vi "保存历史波形图.vi"(4 "接受协议数组":T1(array[cluster]), 6 "Chart legend":T2(array[cluster]), 7 "保存开始":bool, 8 "错误输入":errorcluster, 9 "队列元素":dbl[](array[numeric]), 10 "输入":enum16{"检测按键", "设置路径", "保存数据", "关闭TDMS"}(ring), 11 "tdms file in":refnum<k34>) -> (0 "错误输出":errorcluster, 2 "输出":enum16{"检测按键", "设置路径", "保存数据", "关闭TDMS"}(ring), 3 "tdms file out":refnum<k34>)   [LabVIEW 2016]
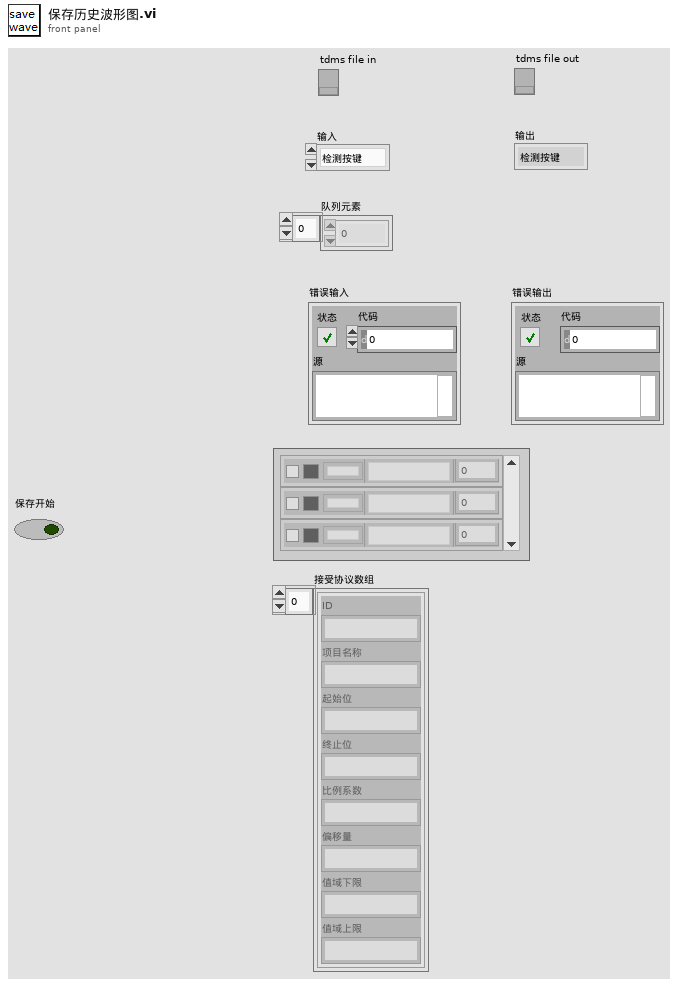
[diagram p1: front panel]
types:
  T1 = cluster{"ID":string, "项目名称":string, "起始位":string, "终止位":string, "比例系数":string, "偏移量":string, "值域下限":string, "值域上限":string}[]
  T2 = cluster{"曲线名称":string, "曲线颜色":u32, "曲线宽度":u16, "当前波形值":dbl, "曲线可见":bool}[]
  T3 = enum16{"open", "open or create", "create or replace", "create", "open (read-only)"}
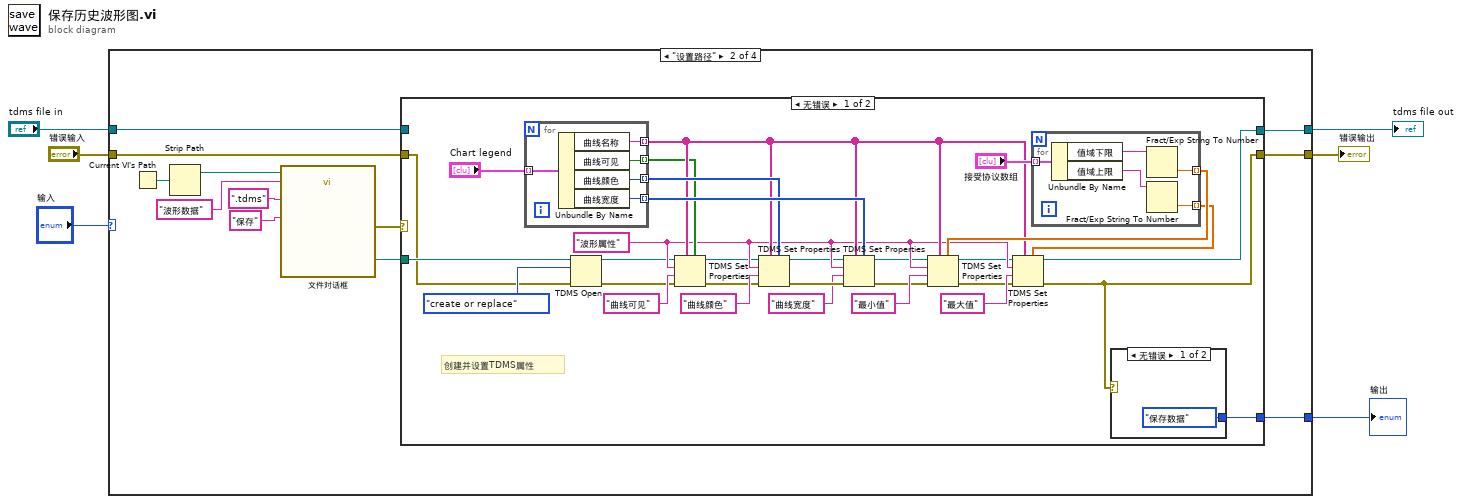
[diagram p0: block diagram]
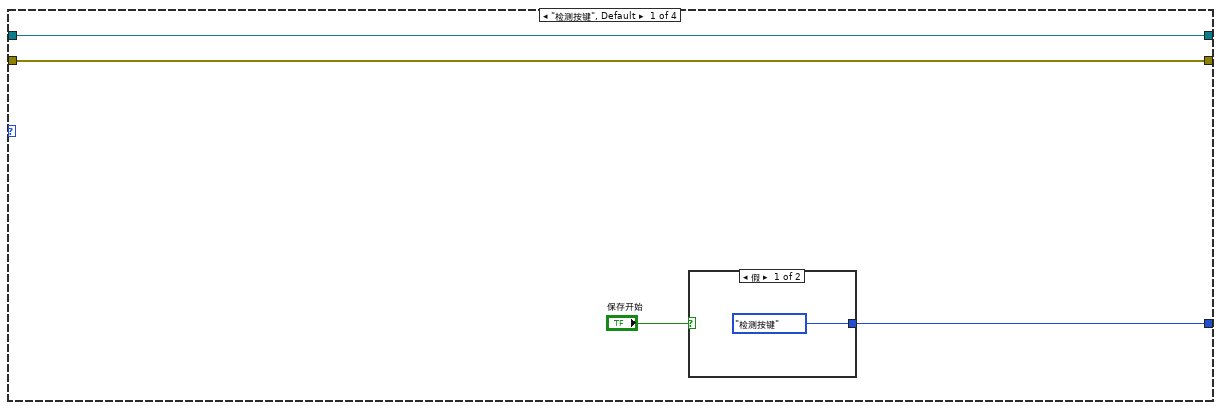
[diagram p2: hidden frame]
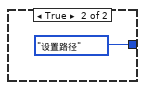
[diagram p3: hidden frame]
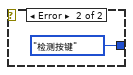
[diagram p4: hidden frame]
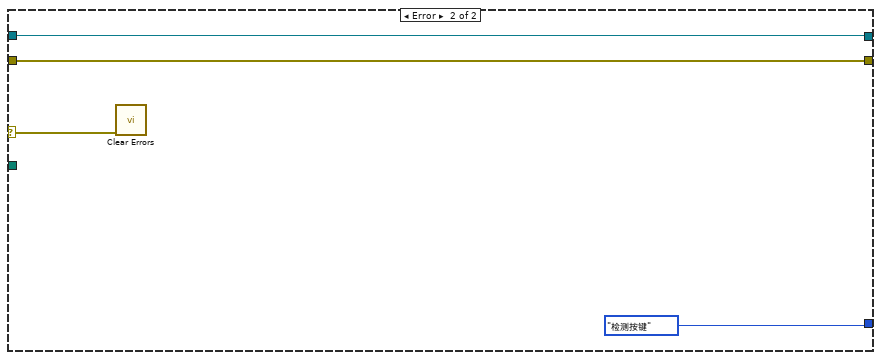
[diagram p5: hidden frame]
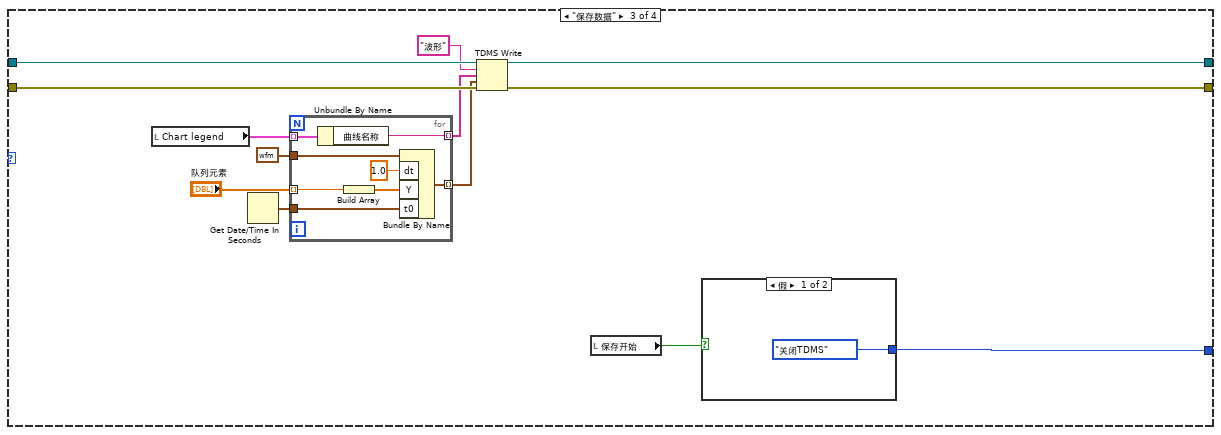
[diagram p6: hidden frame]
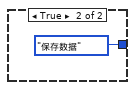
[diagram p7: hidden frame]
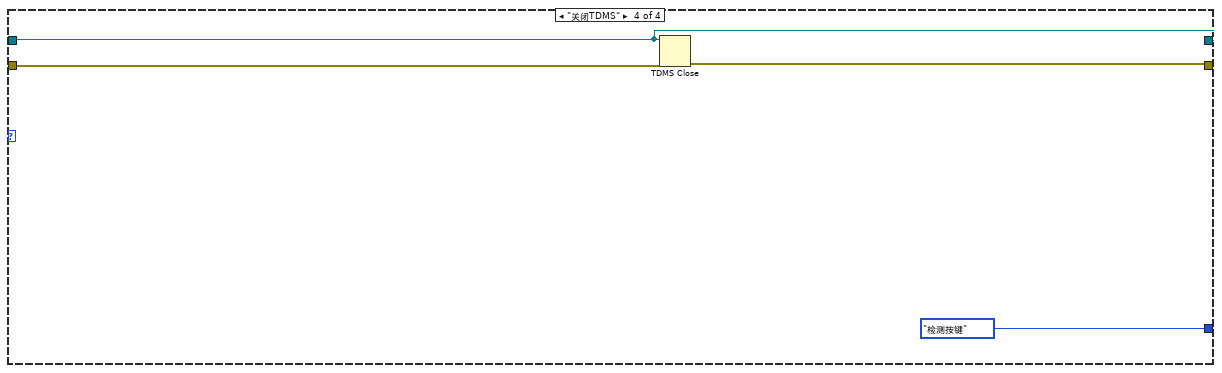
[diagram p8: hidden frame]
diagram:
  n1 = case shown="\"设置路径\"" "输入" {
    tunnel: [w9 w18 w79 enum16{"检测按键", "设置路径", "保存数据", "关闭TDMS"}."检测按键"] -> w5
    tunnel: [w8 w16 w82 w95] -> w1
    tunnel: "tdms file in" -> [w8 w15 w78 w95]
    tunnel: "错误输入" -> [w7 w14 w83 w96]
    tunnel: [w7 w13 w81 w97] -> w4
    frame "检测按键", Default {
      n2 = case shown="假" "保存开始" {
        tunnel: [enum16{"检测按键", "设置路径", "保存数据", "关闭TDMS"}."检测按键" enum16{"检测按键", "设置路径", "保存数据", "关闭TDMS"}."设置路径"] -> w9
        frame False {
        }
        frame True {
        }
      }
    }
    frame "设置路径" {
      n3 = Current VI's Path() -> (path=w24:path)
      n4 = Strip Path(path=w24) -> (stripped path=w20:path)  [unwired: 1 out]
      n5 = call "文件对话框"("start path"=w20, "button label"="保存", "default name"="波形数据", "pattern (all files)"=".tdms") -> ("selected path"=w17:path, "error out"=w19:errorcluster)  [unwired: 8 in, 2 out]
      n6 = case shown="无错误" w19 {
        selector: w19 -> [_ w69]
        tunnel: [w51 enum16{"检测按键", "设置路径", "保存数据", "关闭TDMS"}."检测按键"] -> w18
        tunnel: w17 -> [w53 _]
        tunnel: [w28 w68] -> w16
        tunnel: w15 -> [_ w68]
        tunnel: w14 -> [w52 w67]
        tunnel: [w25 w67] -> w13
        frame No Error {
          w41 = "波形属性" ("组名称")
          # "创建并设置TDMS属性"
          n7 = for {
            tunnel: "Chart legend" -> [w66] mode=indexing
            tunnel: [w65] -> w45 mode=indexing
            tunnel: [w64] -> w44 mode=indexing
            tunnel: [w63] -> w46 mode=indexing
            tunnel: [w62] -> w47 mode=indexing
            n8 = Unbundle By Name(w66) -> ("曲线名称"=w65:string, "曲线可见"=w64:bool, "曲线颜色"=w63:u32, "曲线宽度"=w62:u16)
          }
          n9 = TDMS Open(8:w52, 10:T3."create or replace" ("操作(0:open)"), 11:w53) -> (0:w26:errorcluster, 3:w27:refnum<k34>)  [unwired: 4 in]
          n10 = TDMS Set Properties(5:w44, 7:w45, 8:w26, 9:"曲线可见" ("通道名"), 10:w41, 11:w27) -> (0:w30:errorcluster, 3:w29:refnum<k34>)  [unwired: 2 out]
          n11 = TDMS Set Properties(5:w46, 7:w45, 8:w30, 9:"曲线颜色" ("通道名"), 10:w41, 11:w29) -> (0:w35:errorcluster, 3:w31:refnum<k34>)  [unwired: 2 out]
          n12 = TDMS Set Properties(5:w47, 7:w45, 8:w35, 9:"曲线宽度" ("通道名"), 10:w41, 11:w31) -> (0:w37:errorcluster, 3:w36:refnum<k34>)  [unwired: 2 out]
          n13 = for {
            tunnel: "接受协议数组" -> [w61] mode=indexing
            tunnel: [w58] -> w50 mode=indexing
            tunnel: [w57] -> w49 mode=indexing
            n14 = Unbundle By Name(w61) -> ("值域下限"=w60:string, "值域上限"=w59:string)
            n15 = Fract/Exp String To Number(string=w60) -> (number=w58:dbl)  [unwired: 3 in, 1 out]
            n16 = Fract/Exp String To Number(string=w59) -> (number=w57:dbl)  [unwired: 3 in, 1 out]
          }
          n17 = TDMS Set Properties(5:w50, 7:w45, 8:w37, 9:"最小值" ("通道名"), 10:w41, 11:w36) -> (0:w38:errorcluster, 3:w39:refnum<k34>)  [unwired: 2 out]
          n18 = TDMS Set Properties(5:w49, 7:w45, 8:w38, 9:"最大值" ("通道名"), 10:w41, 11:w39) -> (0:w25:errorcluster, 3:w28:refnum<k34>)  [unwired: 2 out]
          n19 = case shown="无错误" w25 {
            tunnel: [enum16{"检测按键", "设置路径", "保存数据", "关闭TDMS"}."保存数据" enum16{"检测按键", "设置路径", "保存数据", "关闭TDMS"}."检测按键"] -> w51
            frame No Error {
            }
            frame Error {
            }
          }
        }
        frame Error {
          n20 = call <vilib>:"Clear Errors.vi"("error in (no error)"=w69) -> ()  [unwired: 5 in, 2 out]
        }
      }
    }
    frame "保存数据" {
      n21 = local read "Chart legend"() -> (w72:T2)
      n22 = Get Date/Time In Seconds() -> (seconds since 1Jan1904=w77:timestamp)
      n23 = for {
        tunnel: [w91] -> w74 mode=indexing
        tunnel: w77 -> [w90]
        tunnel: [w88] -> w73 mode=indexing
        tunnel: waveform(dbl) {"t0"=timestamp(0 s since 1904-01-01), "dt"=1.0, "Y"=[]} ("波形") -> [w87]
        tunnel: w72 -> [w86] mode=indexing
        tunnel: "队列元素" -> [w85] mode=indexing
        n24 = Unbundle By Name(w86) -> ("曲线名称"=w91:string)
        n25 = Build Array(w85) -> (w84:dbl[])
        n26 = Bundle By Name(cluster=w87, "dt"=1.0, "Y"=w84, "t0"=w90) -> (w88:waveform(dbl))
      }
      n27 = TDMS Write(0:w78, 5:"波形" ("组名称输入（无标题）"), 7:w74, 9:w73, 11:w83) -> (4:w82:refnum<k34>, 15:w81:errorcluster)  [unwired: 1 in, 2 out]
      n28 = local read "保存开始"() -> (w80:bool)
      n29 = case shown="假" w80 {
        tunnel: [enum16{"检测按键", "设置路径", "保存数据", "关闭TDMS"}."关闭TDMS" enum16{"检测按键", "设置路径", "保存数据", "关闭TDMS"}."保存数据"] -> w79
        frame False {
        }
        frame True {
        }
      }
    }
    frame "关闭TDMS" {
      n30 = TDMS Close(8:w96, 11:w95) -> (0:w97:errorcluster)  [unwired: 1 out]
    }
  }
  "输出" <- w5
  "tdms file out" <- w1
  "错误输出" <- w4
